vi "Add Default Free.vi"(8 "error in (no error)":errorcluster, 10 "ToModBus":bool, 11 "Current in":refnum<class "Current.lvclass">) -> (0 "error out":errorcluster, 3 "Current out":refnum<class "Current.lvclass">)   [LabVIEW 2018, in "Measurement Channels.lvlib" / "Current.lvclass"]
uses:
  Current.lvclass
  C:/Users/Jeff Tipps/Documents/DAQMan/source/Classes/Measurements/Class Channel/Channel.lvclass
  Class Channel/Write Unit_EU.vi
  Class Channel/Channel.lvclass
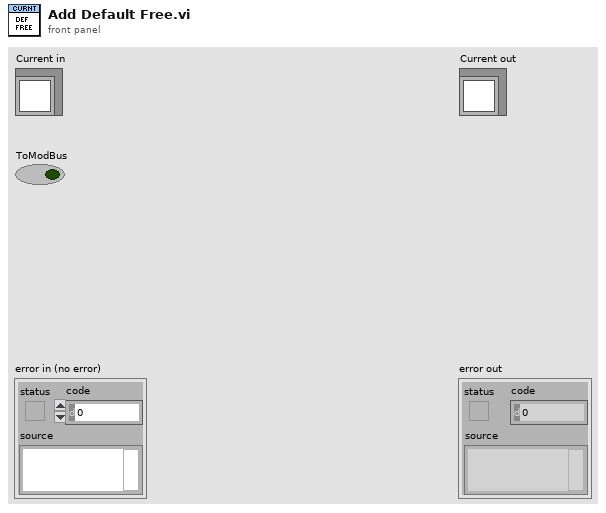
[diagram p1: front panel]
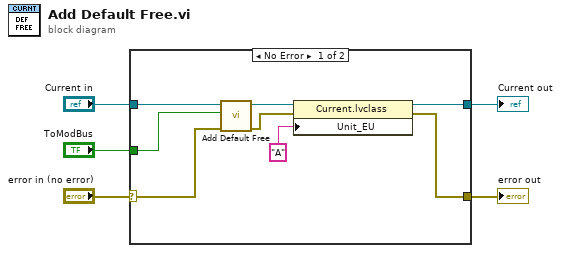
[diagram p0: block diagram]
diagram:
  n1 = case shown="No Error" "error in (no error)" {
    selector: "error in (no error)" -> [w6 w14]
    tunnel: "ToModBus" -> [w13 _]
    tunnel: "Current in" -> [w12 w15]
    tunnel: [w8 w15] -> w3
    tunnel: [w7 w14] -> w2
    frame No Error {
      n2 = call-parent "Add Default Free.vi"("error in (no error)"=w6, "ToModBus"=w13, "Channel in"=w12) -> ("error out"=w10:errorcluster, "Channel out"=w11:refnum<class "Current.lvclass">)  [unwired: 7 in]
      n3 = property class="Current.lvclass"(reference=w11, error in=w10, "Unit_EU"="A") -> (reference out=w8:refnum<class "Current.lvclass">, error out=w7:errorcluster)
    }
    frame Error {
    }
  }
  "error out" <- w2
  "Current out" <- w3
